vi "大舵机加速 (子VI).vi"(10 "数组":bool[](array[boolean]), 11 "PWM输入":dbl) -> (3 "PWM输出 2":dbl)   [LabVIEW 2017, in "年前程序.lvlib"]
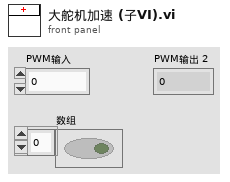
[diagram p1: front panel]
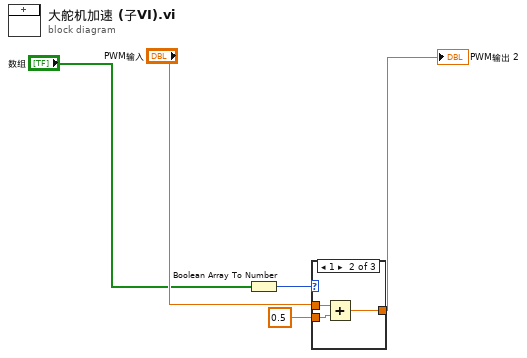
[diagram p0: block diagram]
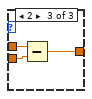
[diagram p3: hidden frame]
diagram:
  n1 = Boolean Array To Number(Boolean array="数组") -> (number=w2:u32)
  n2 = case shown="1" w2 {
    tunnel: "PWM输入" -> [w6 w9 w12]
    tunnel: 0.5 ("y") -> [_ w8 w11]
    tunnel: [w6 w7 w10] -> w4
    frame 0, Default {
    }
    frame 1 {
      n3 = Add(x=w9, y=w8) -> (x+y=w7:dbl)
    }
    frame 2 {
      n4 = Subtract(x=w12, y=w11) -> (x-y=w10:dbl)
    }
  }
  "PWM输出 2" <- w4
